vi "MockHPILC.vi"(11 "MockHPILCSettings":T1={"ModbusRxDataFIFO"="MockbusPort2RxFIFO", "ModbusTxDataFIFO"="MockbusPort2TxFIFO", "BufferUpdateFIFO"="MockHPILCCommand", "Code17Memory"="MockHPILCCode17", "Code18Memory"="MockHPILCCode18", "Code65Memory"="MockHPILCCode65", "Code66Memory"="MockHPILCCode66", "Code67Memory"="MockHPILCCode67", "Code72Memory"="MockHPILCCode72", "Code80Memory"="MockHPILCCode80", "Code110Memory"="MockHPILCCode110", "CRCDataFIFO"="MockHPILCCRCDataFIFO", "CRCCalculateFIFO"="MockHPILCCRCCalculateFIFO", "CRCFIFO"="MockHPILCCRCFIFO"}) -> ()   [LabVIEW 2016, in "FPGAMockHPILC.lvlib"]
uses:
  FPGAMockHPILC.lvlib
  DataTypes/MockHPILCSettings.ctl
  Common_FPGA_Modbus/DataTypes/ModbusCRCSettings.ctl
  Common_FPGA_Modbus/FPGAModbus.lvlib
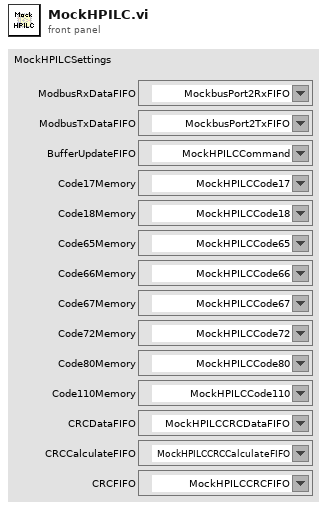
[diagram p1: front panel]
types:
  T1 = typedef "FPGAMockHPILC.lvlib/MockHPILCSettings.ctl" = cluster{"ModbusRxDataFIFO":refnum<k21>, "ModbusTxDataFIFO":refnum<k21>, "BufferUpdateFIFO":refnum<k21>, "Code17Memory":refnum<k21>, "Code18Memory":refnum<k21>, "Code65Memory":refnum<k21>, "Code66Memory":refnum<k21>, "Code67Memory":refnum<k21>, "Code72Memory":refnum<k21>, "Code80Memory":refnum<k21>, "Code110Memory":refnum<k21>, "CRCDataFIFO":refnum<k21>, "CRCCalculateFIFO":refnum<k21>, "CRCFIFO":refnum<k21>}
  T2 = typedef "FPGAModbus.lvlib/ModbusCRCSettings.ctl" = cluster{"DataFIFO":refnum<k21>, "CalculateFIFO":refnum<k21>, "OutputFIFO":refnum<k21>}
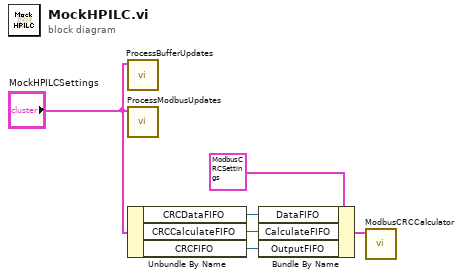
[diagram p0: block diagram]
diagram:
  n1 = call "ProcessBufferUpdates.vi"("MockHPILCSettings"="MockHPILCSettings") -> ()  [unwired: 11 in]
  n2 = call "ProcessModbusUpdates.vi"("MockHPILCSettings"="MockHPILCSettings") -> ()  [unwired: 11 in]
  n3 = Unbundle By Name("MockHPILCSettings") -> ("CRCDataFIFO"=w3:refnum<k21>, "CRCCalculateFIFO"=w2:refnum<k21>, "CRCFIFO"=w1:refnum<k21>)
  n4 = Bundle By Name(cluster=T2 {"DataFIFO"="MockHPILCCRCDataFIFO", "CalculateFIFO"="MockHPILCCRCCalculateFIFO", "OutputFIFO"="MockHPILCCRCFIFO"} ("ModbusCRCSettings"), "DataFIFO"=w3, "CalculateFIFO"=w2, "OutputFIFO"=w1) -> (w5:T2)
  n5 = call "ModbusCRCCalculator.vi"("ModbusCRCSettings"=w5) -> ()  [unwired: 11 in]
